vi "NUM TO ARRAY(SubVI).vi"(1 "A":dbl) -> (0 "Array":dbl[](array[numeric]))   [LabVIEW 2019]
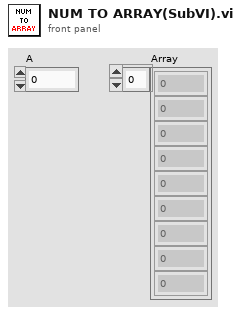
[diagram p1: front panel]
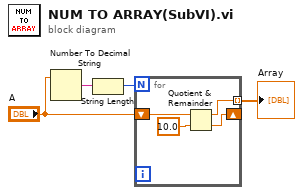
[diagram p0: block diagram]
diagram:
  n1 = Number To Decimal String(number="A") -> (decimal integer string=w2:string)  [unwired: 1 in]
  n2 = String Length(string=w2) -> (length=w1:i32)
  n3 = for {
    N: w1 -> [_]
    shift-right: [w7] -> _
    shift-left: "A" -> [w6]
    tunnel: [w8] -> w4 mode=indexing
    n4 = Quotient & Remainder(x=w6, y=10.0) -> (x-y*floor(x/y)=w8:dbl, floor(x/y)=w7:dbl)
  }
  "Array" <- w4
